vi "Global FPGA.vi"() -> ()   [LabVIEW 2014]
uses:
  <vilib>/Motion/SoftMotion/Synchronization/nism.softmotionScan.timerControl.ctl
  <vilib>/Motion/SoftMotion/Synchronization/nism.softmotionScan.timerConfig.ctl
  <vilib>/Motion/MotorControl/_s/nism.mdo.splineData.ctl
  <vilib>/Motion/MotorControl/_s/nism.splineInterpolation.type.ctl
  <vilib>/Motion/MotorControl/_s/nism.dio.portA.config.2.ctl
  <vilib>/Motion/MotorControl/_s/nism.safeStates.ctl
  <vilib>/Motion/MotorControl/_s/nism.dio.portB.config.2.ctl
  <vilib>/Motion/MotorControl/_s/nism.compare.config.2.ctl
  <vilib>/Motion/MotorControl/_s/nism.compareAction.ctl
  <vilib>/Motion/MotorControl/_s/nism.capture.config.ctl
  <vilib>/Motion/MotorControl/_s/nism.capture.condition.ctl
  <vilib>/Motion/MotorControl/_s/nism.encoder.config.ctl
  <vilib>/Motion/MotorControl/_s/nism.encoder.incremental.config.ctl
  <vilib>/Motion/MotorControl/_s/nism.incremental.indexCriteria.ctl
  <vilib>/Motion/SoftMotion/Synchronization/NI_SoftMotion_Synchronization.lvlib
  <vilib>/Motion/MotorControl/NI_SoftMotion_MotorControlIP.lvlib
panel:
  out "Initialize":bool
  out "Reset I/O":bool
  out "Velocity Filter Active":bool
  out "Encoder Config":T1 caption="encoder config"
  out "DIO Port B Config":T4={"digital filter (us)"=[0, 0, 0, 0, 0, 0, 0, 0], "compare config"={"action"=enum."Pulse", "pulse width"=1, "compare active high?"=TRUE, "window"=0, "safe state"=enum."Low"}, "capture config"={"capture active high?"=FALSE, "position capture condition"=enum."Inactive to Active", "digital filter (ticks)"=2000}, "compare position"=0, "compare period"=0, "safe state"=[enum."Low", enum."Low", enum."Low", enum."Low"]}
  out "DIO Port A Config":T10={"digital filter (us)"=[0, 0, 0, 0, 0, 0, 0, 0], "safe state"=[enum."Low", enum."Low", enum."Low", enum."Low"]}
  out "Index Position":i32 caption="captured position"
  out "Unfiltered Velocity Feedback":i16 caption="xi"
  out "Unfiltered Position Feedback":i32 caption="xi"
  out "Captured Position":i32 caption="captured position"
  out "Minimum Pulse Width (ticks)":u8
  out "Corrected Period":u16
  in  "Index Occurred":bool
  in  "Index Capture Enable":bool
  in  "Current Fault Enable":bool
  out "Drive Enable":bool[](array[boolean])
  in  "Interpolated Position":fxp<+/-,64,32>[](array[numeric])=[0.0, 0.0, 0.0, 0.0, 0.0]
  out "Reset Pending":bool[](array[boolean])
  out "Reset":bool[](array[boolean])
  out "Sync isLocked":bool
  out "Spline Config":T11 caption="spline" {"spline type" items=["cubic b spline", "catmull-rom spline", "linear"]}
  in  "Position Loop Timer Config":T13
  out "Sync isFault":bool
  out "Timer Control":T14 {"sm scan count" format="%x"}
  out "Sync Enable":bool
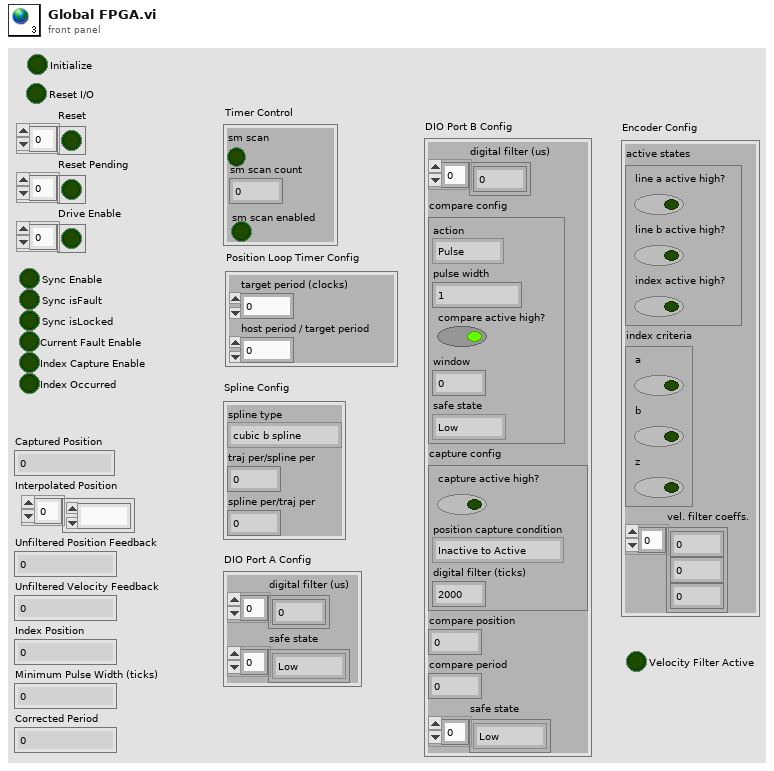
[diagram p1: front panel]
types:
  T1 = typedef "NI_SoftMotion_MotorControlIP.lvlib/nism.encoder.config.ctl" = cluster{"active states":T2, "index criteria":T3, "vel. filter coeffs.":i32[]}
  T2 = typedef "NI_SoftMotion_MotorControlIP.lvlib/nism.encoder.incremental.config.ctl" = cluster{"line a active high?":bool, "line b active high?":bool, "index active high?":bool}
  T3 = typedef "NI_SoftMotion_MotorControlIP.lvlib/nism.incremental.indexCriteria.ctl" = cluster{"a":bool, "b":bool, "z":bool}
  T4 = typedef "NI_SoftMotion_MotorControlIP.lvlib/nism.dio.portB.config.2.ctl" = cluster{"digital filter (us)":u16[], "compare config":T5, "capture config":T8, "compare position":i32, "compare period":i32, "safe state":T7[]}
  T5 = typedef "NI_SoftMotion_MotorControlIP.lvlib/nism.compare.config.2.ctl" = cluster{"action":T6, "pulse width":u16, "compare active high?":bool, "window":i32, "safe state":T7}
  T6 = typedef "NI_SoftMotion_MotorControlIP.lvlib/nism.compareAction.ctl" = enum16{"Pulse", "Toggle", "Set"}
  T7 = typedef "nism.safeStates.ctl" = enum8{"Low", "High", "No Change"}
  T8 = typedef "NI_SoftMotion_MotorControlIP.lvlib/nism.capture.config.ctl" = cluster{"capture active high?":bool, "position capture condition":T9, "digital filter (ticks)":u16}
  T9 = typedef "NI_SoftMotion_MotorControlIP.lvlib/nism.capture.condition.ctl" = enum16{"Inactive to Active", "Active to Inactive"}
  T10 = typedef "NI_SoftMotion_MotorControlIP.lvlib/nism.dio.portA.config.2.ctl" = cluster{"digital filter (us)":u16[], "safe state":T7[]}
  T11 = typedef "NI_SoftMotion_MotorControlIP.lvlib/nism.mdo.splineData.ctl" = cluster{"spline type":T12, "traj per/spline per":u16, "spline per/traj per":fxp<+,32,0>}
  T12 = typedef "NI_SoftMotion_MotorControlIP.lvlib/nism.splineInterpolation.type.ctl" = u16
  T13 = typedef "NI_SoftMotion_Synchronization.lvlib/nism.softmotionScan.timerConfig.ctl" = cluster{"target period (clocks)":u16, "host period / target period":u16}
  T14 = typedef "NI_SoftMotion_Synchronization.lvlib/nism.softmotionScan.timerControl.ctl" = cluster{"sm scan":bool, "sm scan count":u32, "sm scan enabled":bool}
diagram:
